vi "Drive_8CANSwerve.vi"(0 "FrontLeftRotation":dbl, 1 "FrontLeftDrive":dbl, 2 "FrontRightRotation":dbl, 3 "FrontRightDrive":dbl, 4 "RearLeftRotation":dbl, 5 "RearLeftDrive":dbl, 6 "RearRightRotation":dbl, 7 "RearRightDrive":dbl, 11 "PIDInputs":T6, 15 "RotationSettings":T5={"T0"=0, "Mode"=enum."Calibrate", "Rotation Neutral Mode"=enum."Override to Coast", "Rotation Control Mode"=0, "Feedback Device"=8} {"Rotation Control Mode" items=["PercentOutput"=0, "Position"=1, "Velocity"=2, "Current"=3, "Follower"=5, "MotionProfile"=6, "MotionMagic"=7, "MotionProfileArc"=10, "Disabled"=15]; "Feedback Device" items=["QuadEncoder"=0, "Analog"=2, "Tachometer"=4, "Pulse Width Encoded Position"=8, "Sensor Sum (S0 + S1)"=9, "Sensor Difference (D0 - D1)"=10, "Remote Source 0"=11, "Remote Source 1"=12, "Software Emulated"=15]}) -> ()   [LabVIEW 2018]
uses:
  SwerveRotationCalibrate.ctl
  <vilib>/Rock Robotics/WPI/ThirdParty/Phoenix-LabVIEW/Motor Controller/Controls/CTRE_Phoenix_MotorControl_NeutralMode.ctl
  <vilib>/Rock Robotics/WPI/ThirdParty/Phoenix-LabVIEW/Motor Controller/Controls/CTRE_Phoenix_MotorControl_ControlMode.ctl
  <vilib>/Rock Robotics/WPI/ThirdParty/Phoenix-LabVIEW/Motor Controller/Controls/CTRE_Phoenix_MotorControl_FeedbackDevice.ctl
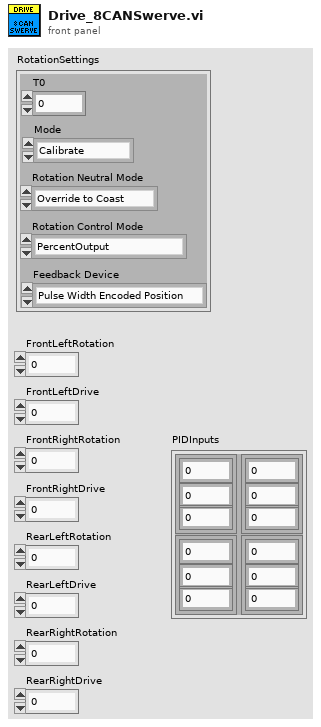
[diagram p1: front panel]
types:
  T1 = typedef "SwerveRotationCalibrate.ctl" = enum16{"Calibrate", "Home", "ManualHome", "ResetQuad", "Drive"}
  T2 = typedef "CTRE_Phoenix_MotorControl_NeutralMode.ctl" = enum8{"EEPROMSetting", "Override to Coast", "Override to Brake"}
  T3 = typedef "CTRE_Phoenix_MotorControl_ControlMode.ctl" = u16
  T4 = typedef "CTRE_Phoenix_MotorControl_FeedbackDevice.ctl" = i8
  T5 = cluster{"T0":u32, "Mode":T1, "Rotation Neutral Mode":T2, "Rotation Control Mode":T3, "Feedback Device":T4}
  T6 = cluster{"Motor1":cluster{"P":dbl, "I":dbl, "D":dbl}, "Motor3":cluster{"P":dbl, "I":dbl, "D":dbl}, "Motor2":cluster{"P":dbl, "I":dbl, "D":dbl}, "Motor4":cluster{"P":dbl, "I":dbl, "D":dbl}}
  T7 = typedef "WPI_MotorControlDeviceRef.ctl" = cluster{"DeviceStatus":errorcluster, "Type":T8, "PWM":cluster{"PWM Channel":T9, "DeadBand":T10}, "CAN":cluster{"Device Number":u8, "SetOutput VI Ref":variant, "GetOutput VI Ref":variant, "Enable VI Ref":variant, "Disable VI Ref":variant, "Data":variant}, "Invert":bool, "DIO PWM":cluster{"PWM \"Enable\" Channel":T9, "DIOChannel":T11, "PWM Rate":dbl}}
  T8 = typedef "WPI_MotorControlType.ctl" = enum16{"PWM", "CAN", "DIO PWM"}
  T9 = typedef "FPGA_DIOPWMChannel.ctl" = enum8{"PWM 0", "PWM 1", "PWM 2", "PWM 3", "PWM 4", "PWM 5", "PWM 6", "PWM 7", "PWM 8", "PWM 9", "PWM MXP 0", "PWM MXP 1", "PWM MXP 2", "PWM MXP 3", "PWM MXP 4", "PWM MXP 5", "PWM MXP 6", "PWM MXP 7", "PWM MXP 8", "PWM MXP 9", "Invalid"}
  T10 = typedef "WPI_PWMDeadband.ctl" = cluster{"Name":string, "maxPositivePwm":i32, "minPositivePwm":i32, "centerPwm":i32, "maxNegativePwm":i32, "minNegativePwm":i32, "angularRange":u16}
  T11 = typedef "FPGA_DIOChannel.ctl" = enum8{"DIO 0", "DIO 1", "DIO 2", "DIO 3", "DIO 4", "DIO 5", "DIO 6", "DIO 7", "DIO 8", "DIO 9", "DIO MXP 0", "DIO MXP 1", "DIO MXP 2", "DIO MXP 3", "DIO MXP 4", "DIO MXP 5", "DIO MXP 6", "DIO MXP 7", "DIO MXP 8", "DIO MXP 9", "DIO MXP 10", "DIO MXP 11", "DIO MXP 12", "DIO MXP 13", "DIO MXP 14", "DIO MXP 15", "SPI Port CS1", "SPI Port CS2", "SPI Port CS3", "SPI Port MISO", "SPI Port MOSI", "Invalid"}
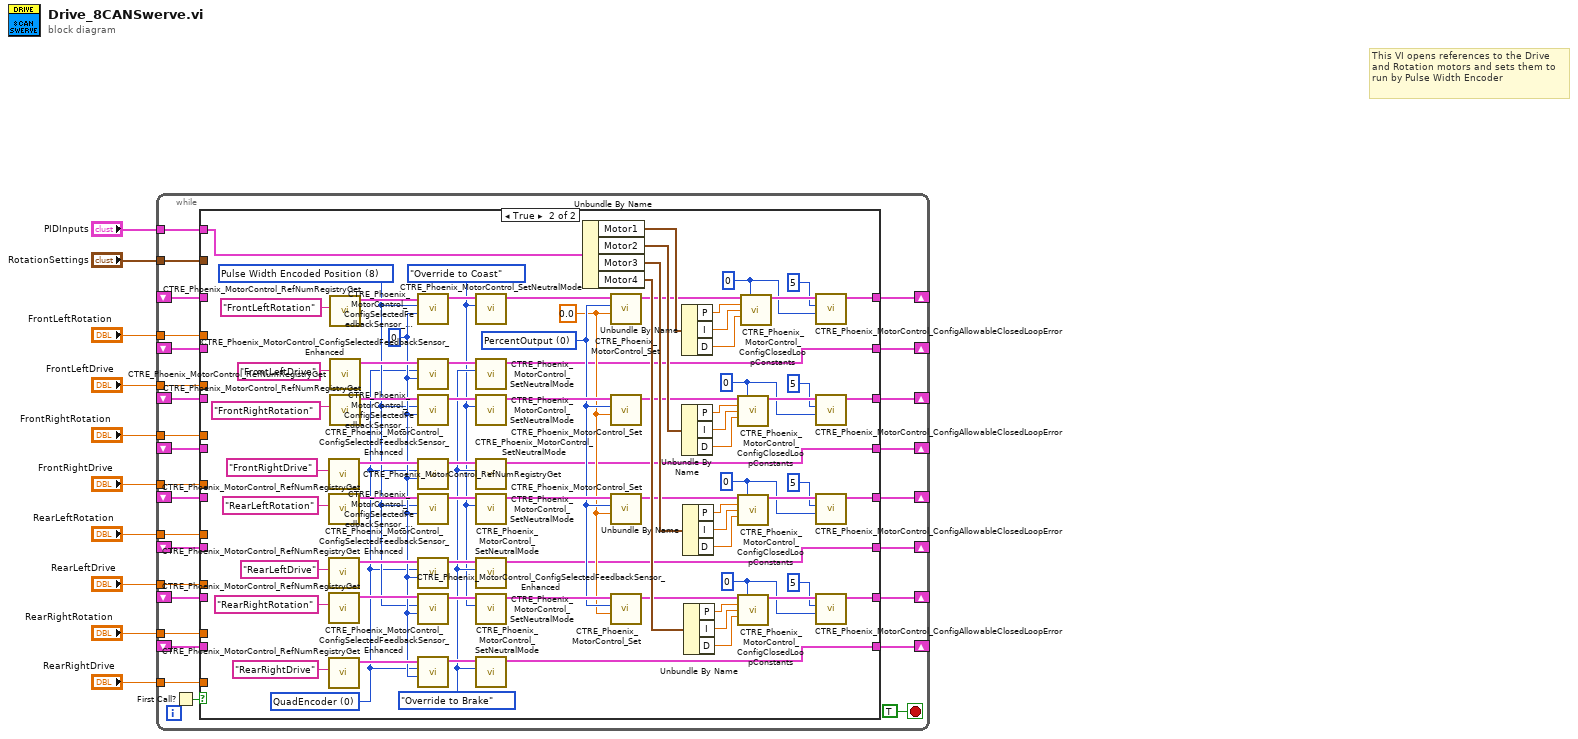
[diagram p0: block diagram]
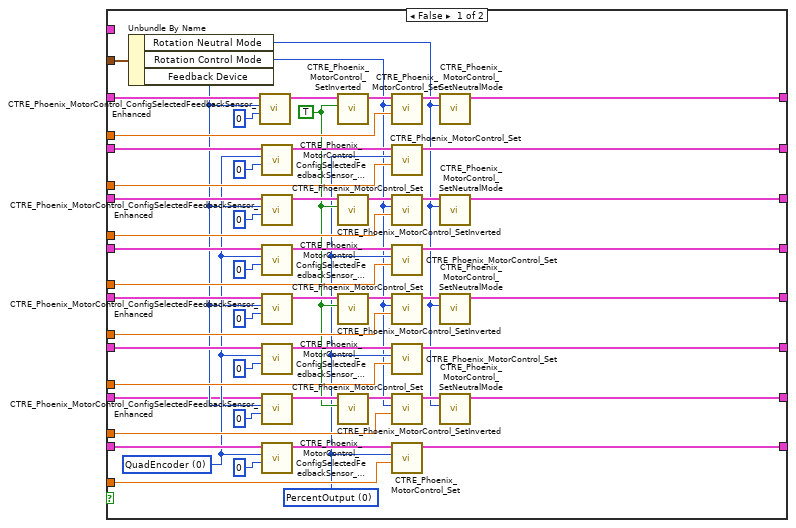
[diagram p2: hidden frame]
diagram:
  # "This VI opens references to the Drive and Rotation motors and sets them to run by Pulse Width Encoder"
  n1 = while {
    shift-right: [w38] -> _
    shift-left: _ -> [w37]
    shift-right: [w15] -> _
    shift-left: _ -> [w35]
    shift-right: [w11] -> _
    shift-left: _ -> [w34]
    shift-right: [w14] -> _
    shift-left: _ -> [w33]
    shift-right: [w36] -> _
    shift-left: _ -> [w32]
    shift-right: [w13] -> _
    shift-left: _ -> [w31]
    shift-right: [w16] -> _
    shift-left: _ -> [w30]
    shift-right: [w12] -> _
    shift-left: _ -> [w29]
    tunnel: "FrontLeftRotation" -> [w26]
    tunnel: "FrontLeftDrive" -> [w25]
    tunnel: "FrontRightRotation" -> [w24]
    tunnel: "FrontRightDrive" -> [w23]
    tunnel: "RearLeftRotation" -> [w22]
    tunnel: "RearLeftDrive" -> [w21]
    tunnel: "RearRightRotation" -> [w20]
    tunnel: "RearRightDrive" -> [w19]
    tunnel: "PIDInputs" -> [w18]
    tunnel: "RotationSettings" -> [w17]
    stop <- TRUE stop-if-true
    n2 = First Call?() -> (First Call?: T/F=w27:bool)
    n3 = case shown="True" w27 {
      tunnel: [w50 w107] -> w38
      tunnel: w37 -> [w71 _]
      tunnel: [w85 w97] -> w15
      tunnel: [w48 w98] -> w11
      tunnel: [w84 w96] -> w14
      tunnel: [w46 w109] -> w36
      tunnel: [w83 w95] -> w13
      tunnel: [w44 w112] -> w16
      tunnel: [w82 w94] -> w12
      tunnel: w35 -> [w72 _]
      tunnel: w34 -> [w73 _]
      tunnel: w33 -> [w70 _]
      tunnel: w32 -> [w69 _]
      tunnel: w31 -> [w68 _]
      tunnel: w30 -> [w39 _]
      tunnel: w29 -> [w67 _]
      tunnel: w26 -> [w93 _]
      tunnel: w25 -> [w92 _]
      tunnel: w24 -> [w91 _]
      tunnel: w23 -> [w90 _]
      tunnel: w22 -> [w89 _]
      tunnel: w21 -> [w88 _]
      tunnel: w20 -> [w87 _]
      tunnel: w19 -> [w86 _]
      tunnel: w18 -> [_ w161]
      tunnel: w17 -> [w40 _]
      frame False {
        w56 = TRUE
        w62 = T4 0 items=["None"=-1, "QuadEncoder"=0, "Analog"=2, "Tachometer"=4, "Pulse Width Encoded Position"=8, "Sensor Sum (S0 + S1)"=9, "Sensor Difference (D0 - D1)"=10, "Remote Source 0"=11, "Remote Source 1"=12, "Software Emulated"=15] ("Feedback Device")
        w52 = T3 0 items=["PercentOutput"=0, "Position"=1, "Velocity"=2, "Current"=3, "Follower"=5, "MotionProfile"=6, "MotionMagic"=7, "MotionMagicArc"=8, "MotionProfileArc"=10, "Disabled"=15] ("Control Mode")
        n4 = Unbundle By Name(w40) -> ("Rotation Neutral Mode"=w41:T2, "Rotation Control Mode"=w42:T3, "Feedback Device"=w43:T4)
        n5 = call <vilib>:"CTRE_Phoenix_MotorControl_ConfigSelectedFeedbackSensor_Enhanced.vi"("pidLoopIdx"=0, "Feedback Device"=w43, "PhoenixMotorControlDevRef"=w71) -> ("PhoenixMotorControlDevRef"=w58:T7)  [unwired: 7 in, 1 out]
        n6 = call <vilib>:"CTRE_Phoenix_MotorControl_ConfigSelectedFeedbackSensor_Enhanced.vi"("pidLoopIdx"=0, "Feedback Device"=w62, "PhoenixMotorControlDevRef"=w72) -> ("PhoenixMotorControlDevRef"=w63:T7)  [unwired: 7 in, 1 out]
        n7 = call <vilib>:"CTRE_Phoenix_MotorControl_ConfigSelectedFeedbackSensor_Enhanced.vi"("pidLoopIdx"=0, "Feedback Device"=w43, "PhoenixMotorControlDevRef"=w73) -> ("PhoenixMotorControlDevRef"=w59:T7)  [unwired: 7 in, 1 out]
        n8 = call <vilib>:"CTRE_Phoenix_MotorControl_ConfigSelectedFeedbackSensor_Enhanced.vi"("pidLoopIdx"=0, "Feedback Device"=w62, "PhoenixMotorControlDevRef"=w70) -> ("PhoenixMotorControlDevRef"=w64:T7)  [unwired: 7 in, 1 out]
        n9 = call <vilib>:"CTRE_Phoenix_MotorControl_ConfigSelectedFeedbackSensor_Enhanced.vi"("pidLoopIdx"=0, "Feedback Device"=w43, "PhoenixMotorControlDevRef"=w69) -> ("PhoenixMotorControlDevRef"=w60:T7)  [unwired: 7 in, 1 out]
        n10 = call <vilib>:"CTRE_Phoenix_MotorControl_ConfigSelectedFeedbackSensor_Enhanced.vi"("pidLoopIdx"=0, "Feedback Device"=w62, "PhoenixMotorControlDevRef"=w68) -> ("PhoenixMotorControlDevRef"=w65:T7)  [unwired: 7 in, 1 out]
        n11 = call <vilib>:"CTRE_Phoenix_MotorControl_ConfigSelectedFeedbackSensor_Enhanced.vi"("pidLoopIdx"=0, "Feedback Device"=w43, "PhoenixMotorControlDevRef"=w39) -> ("PhoenixMotorControlDevRef"=w61:T7)  [unwired: 7 in, 1 out]
        n12 = call <vilib>:"CTRE_Phoenix_MotorControl_ConfigSelectedFeedbackSensor_Enhanced.vi"("pidLoopIdx"=0, "Feedback Device"=w62, "PhoenixMotorControlDevRef"=w67) -> ("PhoenixMotorControlDevRef"=w66:T7)  [unwired: 7 in, 1 out]
        n13 = call <vilib>:"CTRE_Phoenix_MotorControl_SetInverted.vi"("Invert?"=w56, "PhoenixMotorControlDevRef"=w58) -> ("PhoenixMotorControlDevRef"=w57:T7)  [unwired: 8 in, 1 out]
        n14 = call <vilib>:"CTRE_Phoenix_MotorControl_SetInverted.vi"("Invert?"=w56, "PhoenixMotorControlDevRef"=w59) -> ("PhoenixMotorControlDevRef"=w53:T7)  [unwired: 8 in, 1 out]
        n15 = call <vilib>:"CTRE_Phoenix_MotorControl_SetInverted.vi"("Invert?"=w56, "PhoenixMotorControlDevRef"=w60) -> ("PhoenixMotorControlDevRef"=w54:T7)  [unwired: 8 in, 1 out]
        n16 = call <vilib>:"CTRE_Phoenix_MotorControl_SetInverted.vi"("Invert?"=w56, "PhoenixMotorControlDevRef"=w61) -> ("PhoenixMotorControlDevRef"=w55:T7)  [unwired: 8 in, 1 out]
        n17 = call <vilib>:"CTRE_Phoenix_MotorControl_Set.vi"("Output"=w93, "Control Mode"=w42, "PhoenixMotorControlDevRef"=w57) -> ("PhoenixMotorControlDevRef"=w51:T7)  [unwired: 7 in, 1 out]
        n18 = call <vilib>:"CTRE_Phoenix_MotorControl_Set.vi"("Output"=w92, "Control Mode"=w52, "PhoenixMotorControlDevRef"=w63) -> ("PhoenixMotorControlDevRef"=w85:T7)  [unwired: 7 in, 1 out]
        n19 = call <vilib>:"CTRE_Phoenix_MotorControl_Set.vi"("Output"=w91, "Control Mode"=w42, "PhoenixMotorControlDevRef"=w53) -> ("PhoenixMotorControlDevRef"=w49:T7)  [unwired: 7 in, 1 out]
        n20 = call <vilib>:"CTRE_Phoenix_MotorControl_Set.vi"("Output"=w90, "Control Mode"=w52, "PhoenixMotorControlDevRef"=w64) -> ("PhoenixMotorControlDevRef"=w84:T7)  [unwired: 7 in, 1 out]
        n21 = call <vilib>:"CTRE_Phoenix_MotorControl_Set.vi"("Output"=w89, "Control Mode"=w42, "PhoenixMotorControlDevRef"=w54) -> ("PhoenixMotorControlDevRef"=w47:T7)  [unwired: 7 in, 1 out]
        n22 = call <vilib>:"CTRE_Phoenix_MotorControl_Set.vi"("Output"=w88, "Control Mode"=w52, "PhoenixMotorControlDevRef"=w65) -> ("PhoenixMotorControlDevRef"=w83:T7)  [unwired: 7 in, 1 out]
        n23 = call <vilib>:"CTRE_Phoenix_MotorControl_Set.vi"("Output"=w87, "Control Mode"=w42, "PhoenixMotorControlDevRef"=w55) -> ("PhoenixMotorControlDevRef"=w45:T7)  [unwired: 7 in, 1 out]
        n24 = call <vilib>:"CTRE_Phoenix_MotorControl_Set.vi"("Output"=w86, "Control Mode"=w52, "PhoenixMotorControlDevRef"=w66) -> ("PhoenixMotorControlDevRef"=w82:T7)  [unwired: 7 in, 1 out]
        n25 = call <vilib>:"CTRE_Phoenix_MotorControl_SetNeutralMode.vi"("Motor Control Neutral Mode"=w41, "PhoenixMotorControlDevRef"=w51) -> ("PhoenixMotorControlDevRef"=w50:T7)  [unwired: 8 in, 1 out]
        n26 = call <vilib>:"CTRE_Phoenix_MotorControl_SetNeutralMode.vi"("Motor Control Neutral Mode"=w41, "PhoenixMotorControlDevRef"=w49) -> ("PhoenixMotorControlDevRef"=w48:T7)  [unwired: 8 in, 1 out]
        n27 = call <vilib>:"CTRE_Phoenix_MotorControl_SetNeutralMode.vi"("Motor Control Neutral Mode"=w41, "PhoenixMotorControlDevRef"=w47) -> ("PhoenixMotorControlDevRef"=w46:T7)  [unwired: 8 in, 1 out]
        n28 = call <vilib>:"CTRE_Phoenix_MotorControl_SetNeutralMode.vi"("Motor Control Neutral Mode"=w41, "PhoenixMotorControlDevRef"=w45) -> ("PhoenixMotorControlDevRef"=w44:T7)  [unwired: 8 in, 1 out]
      }
      frame True {
        w114 = 0.0 ("Output")
        w115 = T3 0 items=["PercentOutput"=0, "Position"=1, "Velocity"=2, "Current"=3, "Follower"=5, "MotionProfile"=6, "MotionMagic"=7, "MotionProfileArc"=10, "Disabled"=15] ("Control Mode")
        w124 = T4 0 items=["QuadEncoder"=0, "Analog"=2, "Tachometer"=4, "Pulse Width Encoded Position"=8, "Sensor Sum (S0 + S1)"=9, "Sensor Difference (D0 - D1)"=10, "Remote Source 0"=11, "Remote Source 1"=12, "Software Emulated"=15] ("Feedback Device")
        w125 = CTRE_Phoenix_MotorControl_NeutralMode."Override to Coast" ("Motor Control Neutral Mode")
        w126 = CTRE_Phoenix_MotorControl_NeutralMode."Override to Brake" ("Motor Control Neutral Mode")
        w135 = T4 8 items=["QuadEncoder"=0, "Analog"=2, "Tachometer"=4, "Pulse Width Encoded Position"=8, "Sensor Sum (S0 + S1)"=9, "Sensor Difference (D0 - D1)"=10, "Remote Source 0"=11, "Remote Source 1"=12, "Software Emulated"=15] ("Feedback Device")
        w136 = 0 ("pidLoopIdx")
        w111 = 0 ("slotIdx")
        w101 = 0 ("slotIdx")
        w100 = 0 ("slotIdx")
        w99 = 0 ("slotIdx")
        n29 = call <vilib>:"CTRE_Phoenix_MotorControl_RefNumRegistryGet.vi"("refnum name"="FrontRightDrive") -> ("PhoenixMotorControlDevRef"=w142:T7)  [unwired: 9 in, 1 out]
        n30 = call <vilib>:"CTRE_Phoenix_MotorControl_RefNumRegistryGet.vi"("refnum name"="RearLeftRotation") -> ("PhoenixMotorControlDevRef"=w141:T7)  [unwired: 9 in, 1 out]
        n31 = call <vilib>:"CTRE_Phoenix_MotorControl_RefNumRegistryGet.vi"("refnum name"="RearLeftDrive") -> ("PhoenixMotorControlDevRef"=w140:T7)  [unwired: 9 in, 1 out]
        n32 = call <vilib>:"CTRE_Phoenix_MotorControl_RefNumRegistryGet.vi"("refnum name"="RearRightRotation") -> ("PhoenixMotorControlDevRef"=w139:T7)  [unwired: 9 in, 1 out]
        n33 = call <vilib>:"CTRE_Phoenix_MotorControl_RefNumRegistryGet.vi"("refnum name"="RearRightDrive") -> ("PhoenixMotorControlDevRef"=w138:T7)  [unwired: 9 in, 1 out]
        n34 = call <vilib>:"CTRE_Phoenix_MotorControl_RefNumRegistryGet.vi"("refnum name"="FrontLeftRotation") -> ("PhoenixMotorControlDevRef"=w145:T7)  [unwired: 9 in, 1 out]
        n35 = call <vilib>:"CTRE_Phoenix_MotorControl_RefNumRegistryGet.vi"("refnum name"="FrontLeftDrive") -> ("PhoenixMotorControlDevRef"=w144:T7)  [unwired: 9 in, 1 out]
        n36 = call <vilib>:"CTRE_Phoenix_MotorControl_RefNumRegistryGet.vi"("refnum name"="FrontRightRotation") -> ("PhoenixMotorControlDevRef"=w143:T7)  [unwired: 9 in, 1 out]
        n37 = call <vilib>:"CTRE_Phoenix_MotorControl_ConfigSelectedFeedbackSensor_Enhanced.vi"("pidLoopIdx"=w136, "Feedback Device"=w135, "PhoenixMotorControlDevRef"=w145) -> ("PhoenixMotorControlDevRef"=w134:T7)  [unwired: 7 in, 1 out]
        n38 = call <vilib>:"CTRE_Phoenix_MotorControl_ConfigSelectedFeedbackSensor_Enhanced.vi"("pidLoopIdx"=w136, "Feedback Device"=w124, "PhoenixMotorControlDevRef"=w144) -> ("PhoenixMotorControlDevRef"=w132:T7)  [unwired: 7 in, 1 out]
        n39 = call <vilib>:"CTRE_Phoenix_MotorControl_ConfigSelectedFeedbackSensor_Enhanced.vi"("pidLoopIdx"=w136, "Feedback Device"=w135, "PhoenixMotorControlDevRef"=w143) -> ("PhoenixMotorControlDevRef"=w131:T7)  [unwired: 7 in, 1 out]
        n40 = call <vilib>:"CTRE_Phoenix_MotorControl_ConfigSelectedFeedbackSensor_Enhanced.vi"("pidLoopIdx"=w136, "Feedback Device"=w124, "PhoenixMotorControlDevRef"=w142) -> ("PhoenixMotorControlDevRef"=w130:T7)  [unwired: 7 in, 1 out]
        n41 = call <vilib>:"CTRE_Phoenix_MotorControl_ConfigSelectedFeedbackSensor_Enhanced.vi"("pidLoopIdx"=w136, "Feedback Device"=w135, "PhoenixMotorControlDevRef"=w141) -> ("PhoenixMotorControlDevRef"=w133:T7)  [unwired: 7 in, 1 out]
        n42 = call <vilib>:"CTRE_Phoenix_MotorControl_ConfigSelectedFeedbackSensor_Enhanced.vi"("pidLoopIdx"=w136, "Feedback Device"=w124, "PhoenixMotorControlDevRef"=w140) -> ("PhoenixMotorControlDevRef"=w129:T7)  [unwired: 7 in, 1 out]
        n43 = call <vilib>:"CTRE_Phoenix_MotorControl_ConfigSelectedFeedbackSensor_Enhanced.vi"("pidLoopIdx"=w136, "Feedback Device"=w135, "PhoenixMotorControlDevRef"=w139) -> ("PhoenixMotorControlDevRef"=w128:T7)  [unwired: 7 in, 1 out]
        n44 = call <vilib>:"CTRE_Phoenix_MotorControl_ConfigSelectedFeedbackSensor_Enhanced.vi"("pidLoopIdx"=w136, "Feedback Device"=w124, "PhoenixMotorControlDevRef"=w138) -> ("PhoenixMotorControlDevRef"=w127:T7)  [unwired: 7 in, 1 out]
        n45 = call <vilib>:"CTRE_Phoenix_MotorControl_SetNeutralMode.vi"("Motor Control Neutral Mode"=w125, "PhoenixMotorControlDevRef"=w134) -> ("PhoenixMotorControlDevRef"=w121:T7)  [unwired: 8 in, 1 out]
        n46 = call <vilib>:"CTRE_Phoenix_MotorControl_SetNeutralMode.vi"("Motor Control Neutral Mode"=w126, "PhoenixMotorControlDevRef"=w132) -> ("PhoenixMotorControlDevRef"=w97:T7)  [unwired: 8 in, 1 out]
        n47 = call <vilib>:"CTRE_Phoenix_MotorControl_SetNeutralMode.vi"("Motor Control Neutral Mode"=w125, "PhoenixMotorControlDevRef"=w131) -> ("PhoenixMotorControlDevRef"=w119:T7)  [unwired: 8 in, 1 out]
        n48 = call <vilib>:"CTRE_Phoenix_MotorControl_SetNeutralMode.vi"("Motor Control Neutral Mode"=w126, "PhoenixMotorControlDevRef"=w130) -> ("PhoenixMotorControlDevRef"=w96:T7)  [unwired: 8 in, 1 out]
        n49 = call <vilib>:"CTRE_Phoenix_MotorControl_SetNeutralMode.vi"("Motor Control Neutral Mode"=w125, "PhoenixMotorControlDevRef"=w133) -> ("PhoenixMotorControlDevRef"=w117:T7)  [unwired: 8 in, 1 out]
        n50 = call <vilib>:"CTRE_Phoenix_MotorControl_SetNeutralMode.vi"("Motor Control Neutral Mode"=w126, "PhoenixMotorControlDevRef"=w129) -> ("PhoenixMotorControlDevRef"=w95:T7)  [unwired: 8 in, 1 out]
        n51 = call <vilib>:"CTRE_Phoenix_MotorControl_SetNeutralMode.vi"("Motor Control Neutral Mode"=w125, "PhoenixMotorControlDevRef"=w128) -> ("PhoenixMotorControlDevRef"=w123:T7)  [unwired: 8 in, 1 out]
        n52 = call <vilib>:"CTRE_Phoenix_MotorControl_SetNeutralMode.vi"("Motor Control Neutral Mode"=w126, "PhoenixMotorControlDevRef"=w127) -> ("PhoenixMotorControlDevRef"=w94:T7)  [unwired: 8 in, 1 out]
        n53 = Unbundle By Name(w161) -> ("Motor1"=w160:cluster{"P":dbl, "I":dbl, "D":dbl}, "Motor2"=w157:cluster{"P":dbl, "I":dbl, "D":dbl}, "Motor3"=w153:cluster{"P":dbl, "I":dbl, "D":dbl}, "Motor4"=w149:cluster{"P":dbl, "I":dbl, "D":dbl})
        n54 = call <vilib>:"CTRE_Phoenix_MotorControl_Set.vi"("Output"=w114, "Control Mode"=w115, "PhoenixMotorControlDevRef"=w121) -> ("PhoenixMotorControlDevRef"=w120:T7)  [unwired: 7 in, 1 out]
        n55 = call <vilib>:"CTRE_Phoenix_MotorControl_Set.vi"("Output"=w114, "Control Mode"=w115, "PhoenixMotorControlDevRef"=w119) -> ("PhoenixMotorControlDevRef"=w118:T7)  [unwired: 7 in, 1 out]
        n56 = call <vilib>:"CTRE_Phoenix_MotorControl_Set.vi"("Output"=w114, "Control Mode"=w115, "PhoenixMotorControlDevRef"=w117) -> ("PhoenixMotorControlDevRef"=w116:T7)  [unwired: 7 in, 1 out]
        n57 = call <vilib>:"CTRE_Phoenix_MotorControl_Set.vi"("Output"=w114, "Control Mode"=w115, "PhoenixMotorControlDevRef"=w123) -> ("PhoenixMotorControlDevRef"=w122:T7)  [unwired: 7 in, 1 out]
        n58 = Unbundle By Name(w160) -> ("P"=w137:dbl, "I"=w159:dbl, "D"=w158:dbl)
        n59 = Unbundle By Name(w157) -> ("P"=w156:dbl, "I"=w155:dbl, "D"=w154:dbl)
        n60 = Unbundle By Name(w153) -> ("P"=w152:dbl, "I"=w151:dbl, "D"=w150:dbl)
        n61 = Unbundle By Name(w149) -> ("P"=w148:dbl, "I"=w147:dbl, "D"=w146:dbl)
        n62 = call <vilib>:"CTRE_Phoenix_MotorControl_ConfigClosedLoopConstants.vi"("PhoenixMotorControlDevRef"=w118, "slotIdx"=w100, "P"=w156, "I"=w155, "D"=w154) -> ("PhoenixMotorControlDevRef"=w105:T7)  [unwired: 9 in, 1 out]
        n63 = call <vilib>:"CTRE_Phoenix_MotorControl_ConfigClosedLoopConstants.vi"("PhoenixMotorControlDevRef"=w116, "slotIdx"=w101, "P"=w152, "I"=w151, "D"=w150) -> ("PhoenixMotorControlDevRef"=w106:T7)  [unwired: 9 in, 1 out]
        n64 = call <vilib>:"CTRE_Phoenix_MotorControl_ConfigClosedLoopConstants.vi"("PhoenixMotorControlDevRef"=w122, "slotIdx"=w111, "P"=w148, "I"=w147, "D"=w146) -> ("PhoenixMotorControlDevRef"=w113:T7)  [unwired: 9 in, 1 out]
        n65 = call <vilib>:"CTRE_Phoenix_MotorControl_ConfigClosedLoopConstants.vi"("PhoenixMotorControlDevRef"=w120, "slotIdx"=w99, "P"=w137, "I"=w159, "D"=w158) -> ("PhoenixMotorControlDevRef"=w108:T7)  [unwired: 9 in, 1 out]
        n66 = call <vilib>:"CTRE_Phoenix_MotorControl_ConfigAllowableClosedLoopError.vi"("slotIdx"=w99, "allowableClosedLoopError"=5, "PhoenixMotorControlDevRef"=w108) -> ("PhoenixMotorControlDevRef"=w107:T7)  [unwired: 7 in, 1 out]
        n67 = call <vilib>:"CTRE_Phoenix_MotorControl_ConfigAllowableClosedLoopError.vi"("slotIdx"=w100, "allowableClosedLoopError"=5, "PhoenixMotorControlDevRef"=w105) -> ("PhoenixMotorControlDevRef"=w98:T7)  [unwired: 7 in, 1 out]
        n68 = call <vilib>:"CTRE_Phoenix_MotorControl_ConfigAllowableClosedLoopError.vi"("slotIdx"=w101, "allowableClosedLoopError"=5, "PhoenixMotorControlDevRef"=w106) -> ("PhoenixMotorControlDevRef"=w109:T7)  [unwired: 7 in, 1 out]
        n69 = call <vilib>:"CTRE_Phoenix_MotorControl_ConfigAllowableClosedLoopError.vi"("slotIdx"=w111, "allowableClosedLoopError"=5, "PhoenixMotorControlDevRef"=w113) -> ("PhoenixMotorControlDevRef"=w112:T7)  [unwired: 7 in, 1 out]
      }
    }
  }
